vi "PCU_Connect.vi"(0 "GPIBBoard":i32, 1 "Address/ComPort":string, 2 "Communication":T1(ring), 3 "Terminator":enum32{"Cr", "Lf", "CrLf"}(ring), 4 "Portnumber":i32, 5 "error in":errorcluster, 6 "Target":enum32{"rdo100", "rdo110"}(radio), 7 "PCU-100 Control ID":string) -> (14 "Reference out":refnum<k24>, 19 "error out":errorcluster)   [LabVIEW 2017]
uses:
  C:/Users/Ssantec_Test/Documents/GitHub/LV_Instrument_DLL_Sample/DLL/x86/InstrumentDLL.dll
  DLL/x86/InstrumentDLL.dll
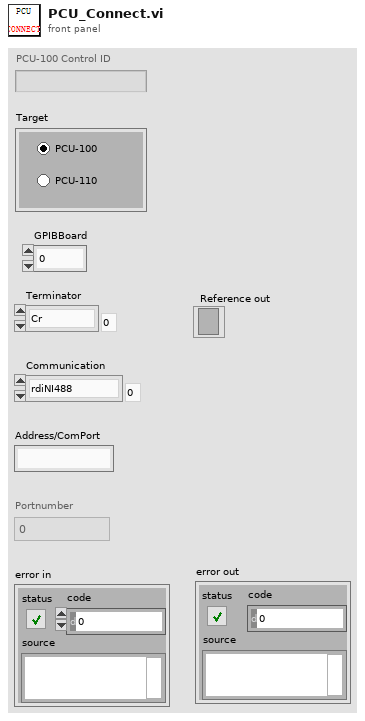
[diagram p1: front panel]
types:
  T1 = enum32{"rdiNI488", "rdiNIvisa", "rdikeysightvisa", "rdiUSB", "rdiLAN"}
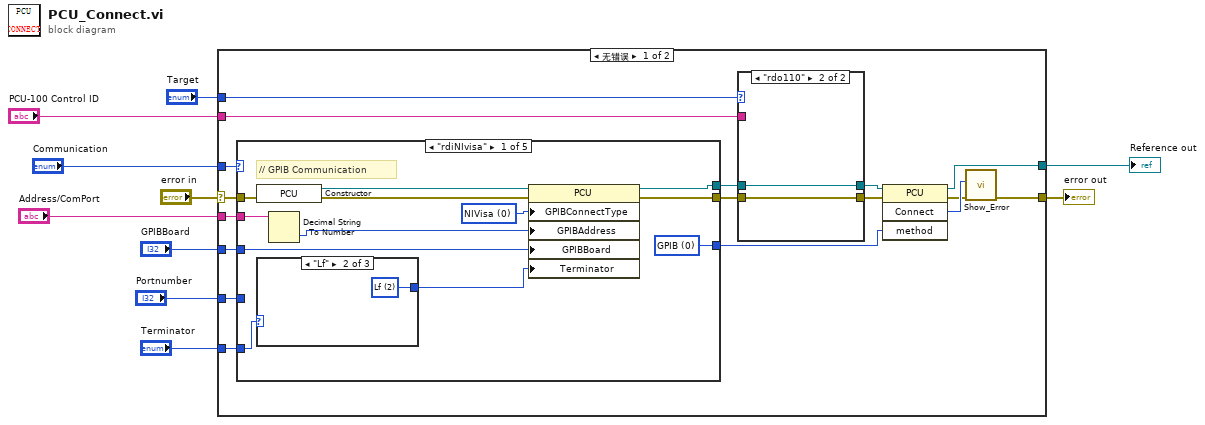
[diagram p0: block diagram]
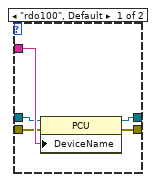
[diagram p2: hidden frame]
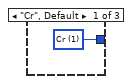
[diagram p3: hidden frame]
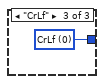
[diagram p4: hidden frame]
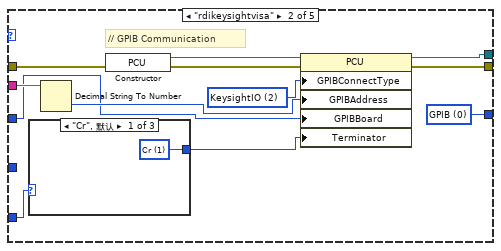
[diagram p5: hidden frame]
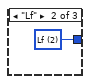
[diagram p6: hidden frame]
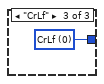
[diagram p7: hidden frame]
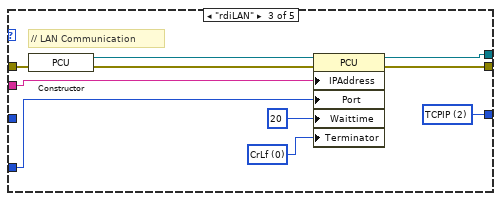
[diagram p8: hidden frame]
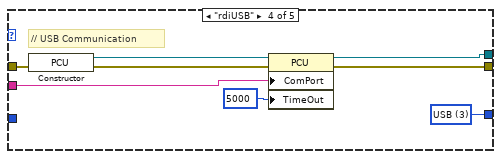
[diagram p9: hidden frame]
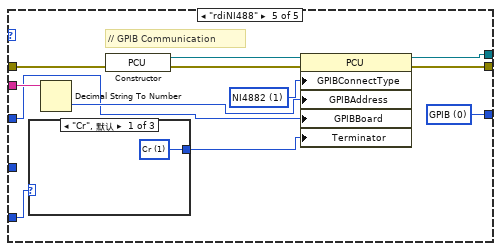
[diagram p10: hidden frame]
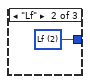
[diagram p11: hidden frame]
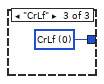
[diagram p12: hidden frame]
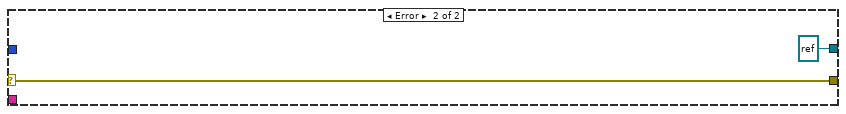
[diagram p13: hidden frame]
diagram:
  n1 = case shown="无错误" "error in" {
    selector: "error in" -> [w24 w99]
    tunnel: "Address/ComPort" -> [w27 _]
    tunnel: [w19 refnum<k24> refnum ("new reference")] -> w9
    tunnel: [w20 w99] -> w8
    tunnel: "Terminator" -> [w26 _]
    tunnel: "Communication" -> [w25 _]
    tunnel: "Portnumber" -> [w18 _]
    tunnel: "GPIBBoard" -> [w17 _]
    tunnel: "Target" -> [w16 _]
    tunnel: "PCU-100 Control ID" -> [w15 _]
    frame No Error {
      n2 = case shown="\"rdiNIvisa\"" w25 {
        tunnel: w27 -> [w44 w59 w74 w80 w92]
        tunnel: w24 -> [w42 w56 w72 w78 w89]
        tunnel: w26 -> [w37 w52 _ _ w85]
        tunnel: [w38 w55 w67 w75 w86] -> w14
        tunnel: [w39 w54 w68 w76 w87] -> w13
        tunnel: [w40 w53 w69 w77 w88] -> w23
        tunnel: w18 -> [_ _ w65 _ _]
        tunnel: w17 -> [w35 w50 _ _ w83]
        frame "rdiNIvisa" {
          w40 = 0 items=["GPIB", "C232C", "TCPIP", "USB"] ("method")
          w46 = 0 items=["NIVisa", "NI4882", "KeysightIO"] ("GPIBConnectType")
          # "// GPIB Communication"
          n3 = constructor class="PCU"(error in=w42) -> (reference out=w43:refnum<k24>, error out=w41:errorcluster)  [unwired: 2 in, 1 out]
          n4 = case shown="\"Lf\"" w37 {
            tunnel: [w47 w48 w49] -> w36
            frame "Cr", Default {
              w47 = 1 items=["CrLf", "Cr", "Lf"] ("Terminator")
            }
            frame "Lf" {
              w48 = 2 items=["CrLf", "Cr", "Lf"] ("Terminator")
            }
            frame "CrLf" {
              w49 = 0 items=["CrLf", "Cr", "Lf"] ("Terminator")
            }
          }
          n5 = Decimal String To Number(string=w44) -> (number=w45:i32)  [unwired: 2 in, 1 out]
          n6 = property on="属性节点" class="PCU"(reference=w43, error in=w41, "GPIBConnectType"=w46, "GPIBAddress"=w45, "GPIBBoard"=w35, "Terminator"=w36) -> (reference out=w38:refnum<k24>, error out=w39:errorcluster)
        }
        frame "rdikeysightvisa" {
          w53 = 0 items=["GPIB", "C232C", "TCPIP", "USB"] ("method")
          w61 = 2 items=["NIVisa", "NI4882", "KeysightIO"] ("GPIBConnectType")
          # "// GPIB Communication"
          n7 = case shown="\"Cr\", 默认" w52 {
            tunnel: [w62 w63 w64] -> w51
            frame "Cr", Default {
              w62 = 1 items=["CrLf", "Cr", "Lf"] ("Terminator")
            }
            frame "Lf" {
              w63 = 2 items=["CrLf", "Cr", "Lf"] ("Terminator")
            }
            frame "CrLf" {
              w64 = 0 items=["CrLf", "Cr", "Lf"] ("Terminator")
            }
          }
          n8 = Decimal String To Number(string=w59) -> (number=w60:i32)  [unwired: 2 in, 1 out]
          n9 = constructor class="PCU"(error in=w56) -> (reference out=w58:refnum<k24>, error out=w57:errorcluster)  [unwired: 2 in, 1 out]
          n10 = property on="属性节点" class="PCU"(reference=w58, error in=w57, "GPIBConnectType"=w61, "GPIBAddress"=w60, "GPIBBoard"=w50, "Terminator"=w51) -> (reference out=w55:refnum<k24>, error out=w54:errorcluster)
        }
        frame "rdiLAN" {
          w66 = 0 items=["CrLf", "Cr", "Lf"] ("Terminator")
          w69 = 2 items=["GPIB", "C232C", "TCPIP", "USB"] ("method")
          # "// LAN Communication"
          n11 = constructor class="PCU"(error in=w72) -> (reference out=w73:refnum<k24>, error out=w71:errorcluster)  [unwired: 2 in, 1 out]
          n12 = property on="属性节点" class="PCU"(reference=w73, error in=w71, "IPAddress"=w74, "Port"=w65, "Waittime"=20, "Terminator"=w66) -> (reference out=w67:refnum<k24>, error out=w68:errorcluster)
        }
        frame "rdiUSB" {
          w77 = 3 items=["GPIB", "C232C", "TCPIP", "USB"] ("method")
          # "// USB Communication"
          n13 = constructor class="PCU"(error in=w78) -> (reference out=w82:refnum<k24>, error out=w79:errorcluster)  [unwired: 2 in, 1 out]
          n14 = property on="属性节点" class="PCU"(reference=w82, error in=w79, "ComPort"=w80, "TimeOut"=5000 ("BaudRate")) -> (reference out=w75:refnum<k24>, error out=w76:errorcluster)
        }
        frame "rdiNI488" {
          w88 = 0 items=["GPIB", "C232C", "TCPIP", "USB"] ("method")
          w94 = 1 items=["NIVisa", "NI4882", "KeysightIO"] ("GPIBConnectType")
          # "// GPIB Communication"
          n15 = case shown="\"Cr\", 默认" w85 {
            tunnel: [w95 w96 w97] -> w84
            frame "Cr", Default {
              w95 = 1 items=["CrLf", "Cr", "Lf"] ("Terminator")
            }
            frame "Lf" {
              w96 = 2 items=["CrLf", "Cr", "Lf"] ("Terminator")
            }
            frame "CrLf" {
              w97 = 0 items=["CrLf", "Cr", "Lf"] ("Terminator")
            }
          }
          n16 = Decimal String To Number(string=w92) -> (number=w93:i32)  [unwired: 2 in, 1 out]
          n17 = constructor class="PCU"(error in=w89) -> (reference out=w91:refnum<k24>, error out=w90:errorcluster)  [unwired: 2 in, 1 out]
          n18 = property on="属性节点" class="PCU"(reference=w91, error in=w90, "GPIBConnectType"=w94, "GPIBAddress"=w93, "GPIBBoard"=w83, "Terminator"=w84) -> (reference out=w86:refnum<k24>, error out=w87:errorcluster)
        }
      }
      n19 = case shown="\"rdo110\"" w16 {
        tunnel: w15 -> [w32 _]
        tunnel: w14 -> [w31 w34]
        tunnel: w13 -> [w30 w33]
        tunnel: [w29 w34] -> w12
        tunnel: [w28 w33] -> w11
        frame "rdo100", Default {
          n20 = property on="属性节点" class="PCU"(reference=w31, error in=w30, "DeviceName"=w32) -> (reference out=w29:refnum<k24>, error out=w28:errorcluster)
        }
        frame "rdo110" {
        }
      }
      n21 = invoke on="调用节点" class="PCU" method="Connect"(reference=w12, error in=w11, "method"=w23) -> (reference out=w19:refnum<k24>, error out=w21:errorcluster, "Connect"=w22:i32)  [unwired: 1 in, 1 out]
      n22 = call "Show_Error.vi"("error in (no error)"=w21, "Error"=w22) -> ("error out"=w20:errorcluster)  [unwired: 9 in]
    }
    frame Error {
    }
  }
  "Reference out" <- w9
  "error out" <- w8
